vi "Instantiate_llm_anthropic.vi"(0 "model_name":string(combo)="claude-3-5-sonnet-20240620", 5 "anthropic_version":string="2023-06-01", 7 "anthropic_key":string, 11 "error in (no error)":errorcluster) -> (4 "llm_anthropic_chatmodels out":refnum<class "llm_anthropic_chatmodels.lvclass">, 15 "error out":errorcluster)   [LabVIEW 2020, in "llm_anthropic_chatmodels.lvclass"]
uses:
  llm_anthropic_chatmodels.lvclass
  D:/Personal/LabVIEW LLMs/src/models/abstract_llm_base/abstract_llm_base.lvclass
  llm_anthropic_chatmodels.lvclass/llm_anthropic_chatmodels.ctl
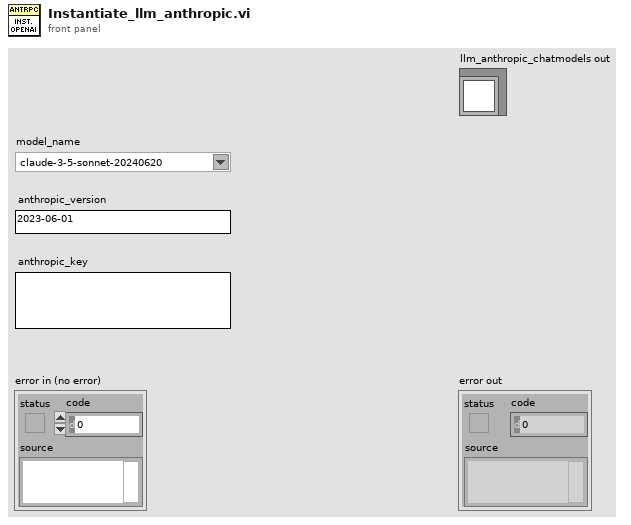
[diagram p1: front panel]
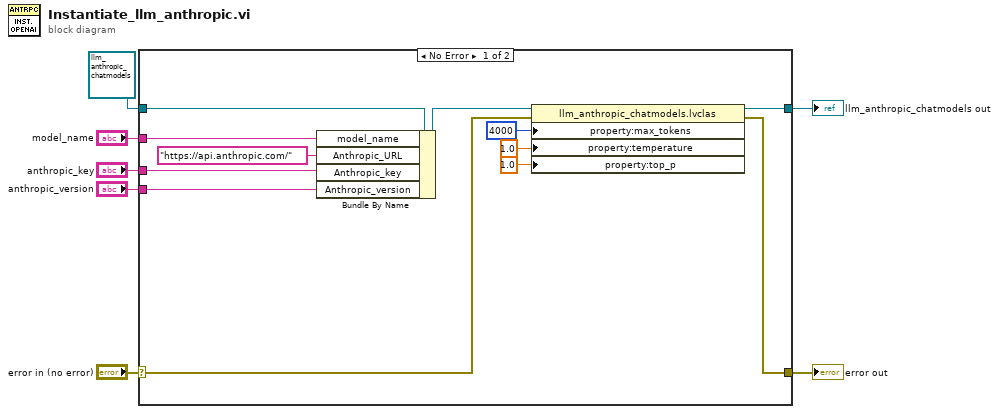
[diagram p0: block diagram]
diagram:
  n1 = case shown="No Error" "error in (no error)" {
    selector: "error in (no error)" -> [w13 w21]
    tunnel: [w12 w21] -> w6
    tunnel: [w14 w20] -> w4
    tunnel: refnum<class "llm_anthropic_chatmodels.lvclass"> refnum ("llm_anthropic_chatmodels in") -> [w19 w20]
    tunnel: "model_name" -> [w18 _]
    tunnel: "anthropic_key" -> [w16 _]
    tunnel: "anthropic_version" -> [w8 _]
    frame No Error {
      n2 = Bundle By Name(cluster=w19, "model_name"=w18, "Anthropic_URL"="https://api.anthropic.com/" ("OpenAI_URL"), "Anthropic_key"=w16, "Anthropic_version"=w8) -> (w15:refnum<class "llm_anthropic_chatmodels.lvclass">)
      n3 = property class="llm_anthropic_chatmodels.lvclas"(reference=w15, error in=w13, "property:max_tokens"=u32 4000 ("max_tokens"), "property:temperature"=1.0 ("temperature"), "property:top_p"=1.0 ("top_p")) -> (reference out=w14:refnum<class "llm_anthropic_chatmodels.lvclass">, error out=w12:errorcluster)
    }
    frame Error {
    }
  }
  "error out" <- w6
  "llm_anthropic_chatmodels out" <- w4
